vi "FinalizeHWI.vi"(8 "error in (no error)":errorcluster, 10 "Master Device in":refnum<class "Master Device.lvclass">, 11 "Arduino in":refnum<class "Arduino.lvclass">) -> (0 "error out":errorcluster, 2 "Master Device out":refnum<class "Master Device.lvclass">, 3 "Arduino out":refnum<class "Arduino.lvclass">)   [LabVIEW 2013, in "Arduino.lvclass"]
uses:
  Arduino.lvclass
  Master Device/Master Device.lvclass
  Arduino.lvclass/Arduino.ctl
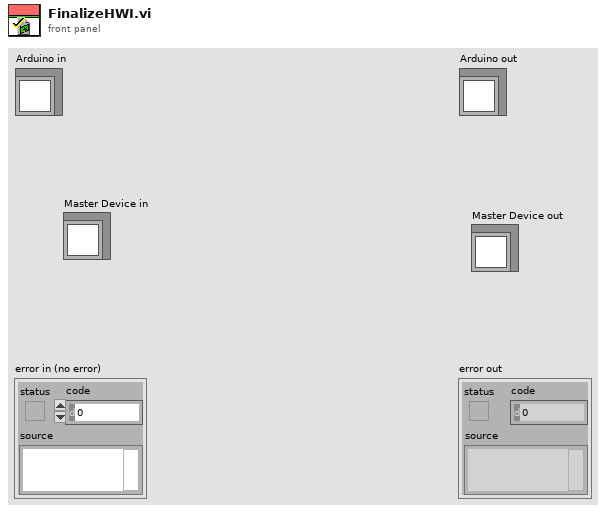
[diagram p1: front panel]
types:
  T1 = cluster{"Short Command":string, "ParamTotal":dbl, "Params":dbl[]}[][]
  T2 = cluster{"Short Command":string, "ParamTotal":dbl, "Params":dbl[]}[]
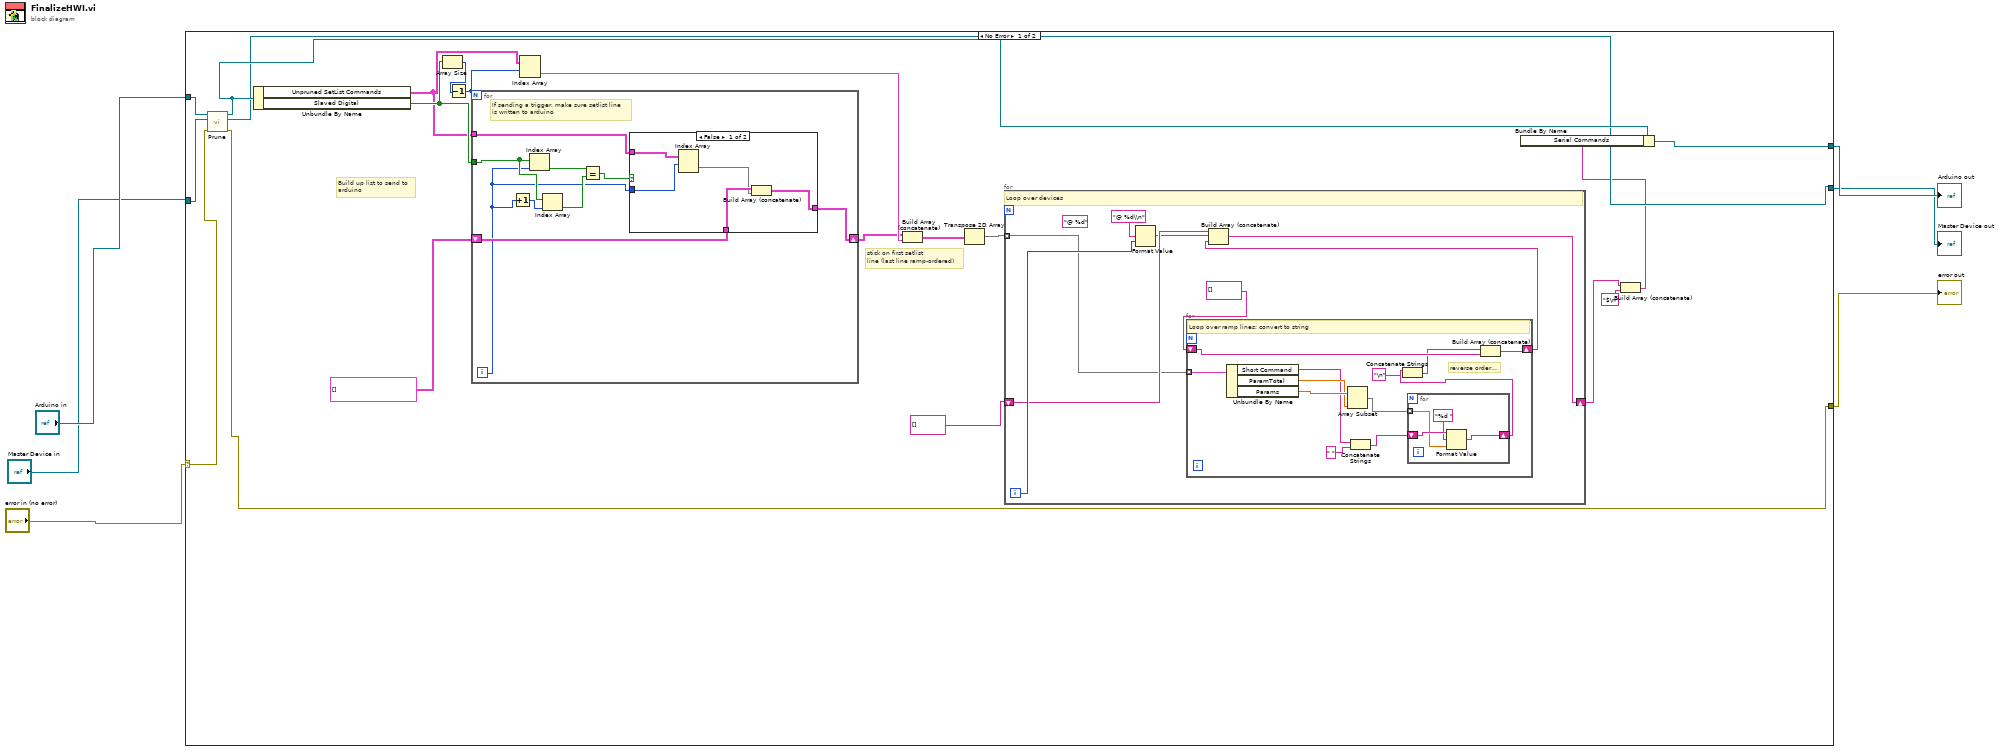
[diagram p0: block diagram]
diagram:
  n1 = case shown="No Error" "error in (no error)" {
    selector: "error in (no error)" -> [w13 w68]
    tunnel: [w10 w68] -> w4
    tunnel: [w11 w67] -> w5
    tunnel: "Master Device in" -> [w14 w67]
    tunnel: [w22 w66] -> w6
    tunnel: "Arduino in" -> [w15 w66]
    frame No Error {
      # "stick on first setlist\nline (last line ramp-ordered)"
      # "Build up list to send to\narduino"
      n2 = call-dynamic "Prune.vi"("error in (no error)"=w13, "Master Device in"=w14, "Arduino in"=w15) -> ("error out"=w10:errorcluster, "Master Device out"=w11:refnum<class "Master Device.lvclass">, "Arduino out"=w12:refnum<class "Arduino.lvclass">)  [unwired: 6 in]
      n3 = Unbundle By Name(w12) -> ("Unpruned SetList Commands"=w20:T1, "Slaved Digital"=w25:bool[])
      n4 = Array Size(array=w25) -> (size(s)=w21:i32)
      n5 = Decrement(x=w21) -> (x-1=w19:i32)
      n6 = for {
        N: w19 -> [_]
        tunnel: w20 -> [w52]
        tunnel: w25 -> [w58]
        shift-right: [w54] -> w17
        shift-left: T1 [] ("Unpruned SetList Commands") -> [w53]
        i -> [w51]
        # "If sending a trigger, make sure setlist line\nis written to arduino"
        n7 = Increment(x=w51) -> (x+1=w59:i32)
        n8 = Index Array(array=w58, index=w51) -> (element=w57:bool)
        n9 = Index Array(array=w58, index=w59) -> (element=w56:bool)
        n10 = Equal?(x=w57, y=w56) -> (x = y?=w55:bool)
        n11 = case shown="False" w55 {
          tunnel: [w63 w65] -> w54
          tunnel: w53 -> [w64 w65]
          tunnel: w52 -> [w62 _]
          tunnel: w51 -> [w61 _]
          frame False {
            n12 = Index Array(array=w62, index (row)=w61) -> (element=w60:T2)  [unwired: 1 in]
            n13 = Build Array (concatenate)(w64, w60) -> (w63:T1)
          }
          frame True {
          }
        }
      }
      n14 = Index Array(array=w20, index (row)=w19) -> (element=w18:T2)  [unwired: 1 in]
      n15 = Build Array (concatenate)(w17, w18) -> (w16:T1)
      n16 = Transpose 2D Array(2D array=w16) -> (transposed array=w24:T1)
      n17 = for {
        tunnel: w24 -> [w31] mode=indexing
        shift-right: [w28] -> w9
        shift-left: string[] [] -> [w33]
        i -> [w34]
        (unwired) "@ %d"
        # "Loop over devices"
        n18 = Format Value(format string="@ %d\\n", value (0)=w34) -> (output string=w32:string)  [unwired: 1 in]
        n19 = for {
          tunnel: w31 -> [w46] mode=indexing
          shift-right: [w41] -> w29
          shift-left: string[] [] ("appended array") -> [w38]
          # "reverse order..."
          # "Loop over ramp lines; convert to string"
          n20 = Unbundle By Name(w46) -> ("Short Command"=w43:string, "ParamTotal"=w44:dbl, "Params"=w45:dbl[])
          n21 = Array Subset(array=w45, length=w44) -> (w40:dbl[])  [unwired: 1 in]
          n22 = Concatenate Strings(w43, " ") -> (w39:string)
          n23 = for {
            tunnel: w40 -> [w48] mode=indexing
            shift-right: [w47] -> w37
            shift-left: w39 -> [w50]
            n24 = Format Value(string ("")=w50, format string="%d ", value (0)=w48) -> (output string=w47:string)
          }
          n25 = Concatenate Strings(w37, "\n") -> (w36:string)
          n26 = Build Array (concatenate)(w36, w38) -> (w41:string[])
        }
        n27 = Build Array (concatenate)(w33, w32, w29) -> (w28:string[])
      }
      n28 = Build Array (concatenate)(w9, "$\n") -> (w7:string[])
      n29 = Bundle By Name(cluster=w12, "Serial Commands"=w7) -> (w22:refnum<class "Arduino.lvclass">)
    }
    frame Error {
    }
  }
  "error out" <- w4
  "Arduino out" <- w6
  "Master Device out" <- w5
